vi "Review Intermediate Result.vi"(0 "Vector 26GHz Path in":refnum<class "Vector Path.lvclass">, 5 "One-Port Charact Data In":T1, 11 "error in (no error)":errorcluster) -> (4 "Vector 26GHz Path out":refnum<class "Vector Path.lvclass">, 6 "Response":string, 8 "One-Port Charact Data Out":T1, 15 "error out":errorcluster)   [LabVIEW 2023, in "RFFixtureCharact.Public.lvlib" / "Vector Path.lvclass"]
uses:
  Vector Path.lvclass
  C:/rfcal/AuxTools/STSRFFixtureCharactUtility/Source/Code Modules/Common/Base Classes/Path/Path.lvclass
  Instruments/Cal Standard/Type Definitions/One-Port Charact Data.ctl
  Instruments/Cal Standard/Type Definitions/Standard Type.ctl
  <vilib>/Utility/error.llb/Trim Whitespace One-Sided.vi
  Vector Path.lvclass/Vector Path.ctl
  Vector Abstract Path/Vector Abstract Path.lvclass
  Common/RFCalAndFixtureCharact.Common.lvlib
  Instruments/RFFixtureCharact.Instruments.lvlib
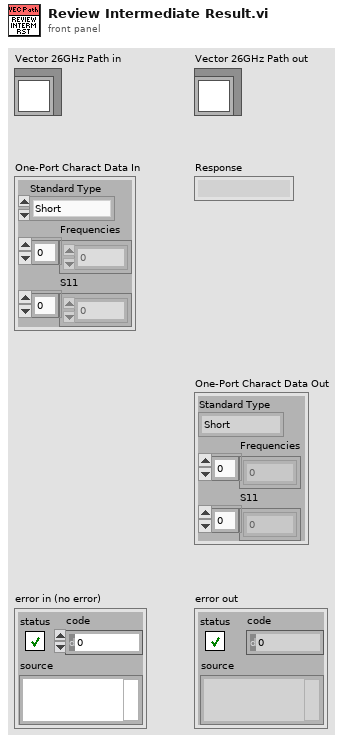
[diagram p1: front panel]
types:
  T1 = typedef "RFFixtureCharact.Instruments.lvlib/One-Port Charact Data.ctl" = cluster{"Standard Type":T2, "Frequencies":dbl[], "S11":cdb[]}
  T2 = typedef "RFFixtureCharact.Instruments.lvlib/Standard Type.ctl" = enum16{"Short", "Open", "Load", "PowerMeter", "None"}
  T3 = typedef "RFFixtureCharact.Public.lvlib/Vector Path Group.lvclass/Sweep.ctl" = cluster{"Port Power":dbl, "Frequencies":dbl[], "Test Receiver Attenuation":dbl, "IF Bandwidth":dbl}
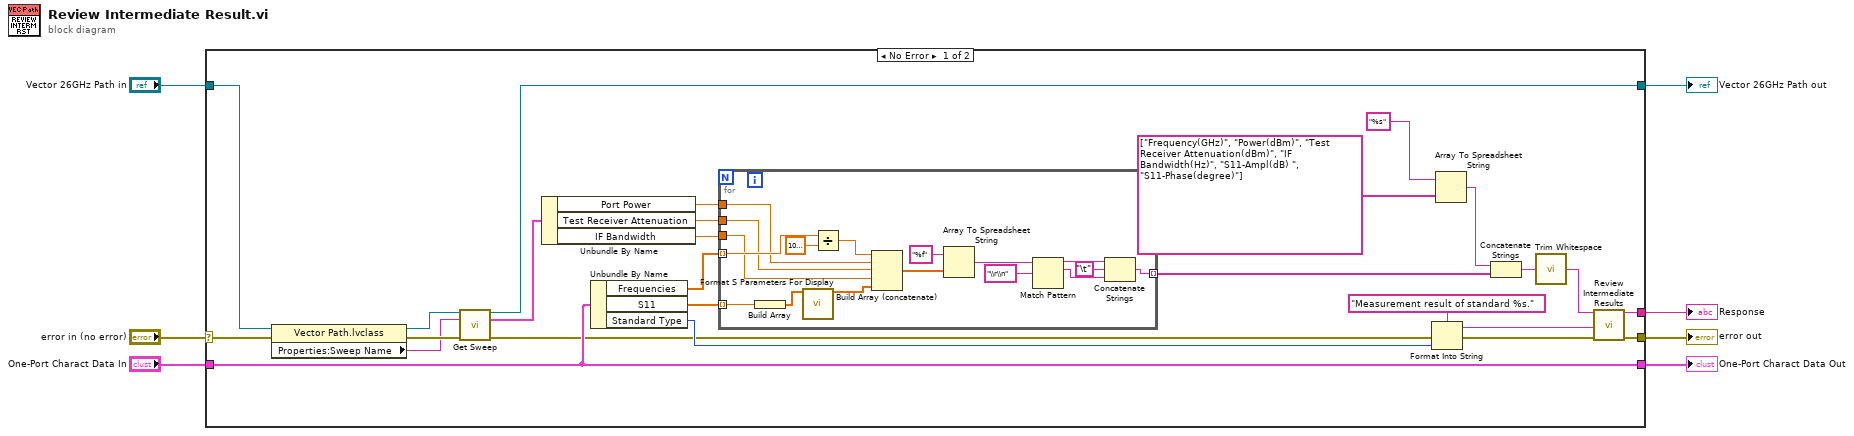
[diagram p0: block diagram]
diagram:
  n1 = case shown="No Error" "error in (no error)" {
    selector: "error in (no error)" -> [w17 w52]
    tunnel: [w24 w52] -> w6
    tunnel: [w25 _] -> w4
    tunnel: [w13 _] -> w5
    tunnel: "Vector 26GHz Path in" -> [w19 w51]
    tunnel: [w8 w51] -> w2
    tunnel: "One-Port Charact Data In" -> [w13 _]
    frame No Error {
      n2 = property class="Vector Path.lvclass"(reference=w19, error in=w17) -> (reference out=w10:refnum<class "Vector Path.lvclass">, error out=w18:errorcluster, "Properties:Sweep Name"=w11:string)
      n3 = call-dynamic "Get Sweep.vi"("Vector Path in"=w10, "Sweep Name"=w11, "error in (no error)"=w18) -> ("Vector Path out"=w8:refnum<class "Vector Path.lvclass">, "Sweep"=w9:T3, "error out"=w12:errorcluster)  [unwired: 9 in, 1 out]
      n4 = Unbundle By Name(w9) -> ("Port Power"=w16:dbl, "Test Receiver Attenuation"=w15:dbl, "IF Bandwidth"=w14:dbl)
      n5 = Unbundle By Name(w13) -> ("Frequencies"=w27:dbl[], "S11"=w28:cdb[], "Standard Type"=w21:T2)
      n6 = for {
        tunnel: [w41] -> w30 mode=indexing
        tunnel: w28 -> [w39] mode=indexing
        tunnel: w27 -> [w37] mode=indexing
        tunnel: w16 -> [w36]
        tunnel: w14 -> [w34]
        tunnel: w15 -> [w35]
        n7 = Build Array(w39) -> (w38:cdb[])
        n8 = call "Format S Parameters For Display.vi"("S Parameters"=w38) -> ("S Parameters For Display"=w40:dbl[])  [unwired: 14 in]
        n9 = Divide(x=w37, y=1000000000.0) -> (x/y=w49:dbl)
        n10 = Build Array (concatenate)(w49, w36, w35, w34, w40) -> (w45:dbl[])
        n11 = Array To Spreadsheet String(array=w45, 3:"%f" ("format string")) -> (spreadsheet string=w47:string)  [unwired: 1 in]
        n12 = Match Pattern(string=w47, regular expression="\\r\\n") -> (before substring=w44:string, match substring=w42:string)  [unwired: 1 in, 2 out]
        n13 = Concatenate Strings(w44, "\t", w42) -> (w41:string)
      }
      n14 = Format Into String(format string="Measurement result of standard %s." ("Request Header"), error in=w12, w21) -> (resulting string=w20:string, error out=w23:errorcluster)  [unwired: 1 in]
      n15 = Array To Spreadsheet String(array=string[] ["Frequency(GHz)", "Power(dBm)", "Test Receiver Attenuation(dBm)", "IF Bandwidth(Hz)", "S11-Ampl(dB) ", "S11-Phase(degree)"], 3:"%s" ("format string")) -> (spreadsheet string=w31:string)  [unwired: 1 in]
      n16 = Concatenate Strings(w31, w30) -> (w29:string)
      n17 = call <vilib>:"Trim Whitespace.vi"("string"=w29) -> ("trimmed string"=w26:string)  [unwired: 1 in]
      n18 = call "Review Intermediate Results.vi"("Intermediate Results"=w26, "Request Header"=w20, "error in (no error)"=w23) -> ("Response"=w25:string, "error out"=w24:errorcluster)  [unwired: 11 in]
    }
    frame Error {
    }
  }
  "error out" <- w6
  "Vector 26GHz Path out" <- w2
  "Response" <- w4
  "One-Port Charact Data Out" <- w5
